vi "Global.vi"() -> ()   [LabVIEW 2020]
panel:
  in  "产品型号":string
  in  "结果显示字":refnum<vi>
  in  "前序状态显示字":refnum<vi>
  in  "前序状态":refnum<vi>
  in  "检测结果":refnum<vi>
  in  "合格数量":refnum<vi>
  in  "生产数量":refnum<vi>
  out "模式":u32
  in  "更换产品":refnum<vi>
  in  "提示信息":refnum<vi>
  in  "程序自动":refnum<vi>
  in  "报警图标":refnum<vi>
  in  "程序关闭":bool
  in  "Info":refnum<vi>
  in  "Result":refnum<vi>
  in  "批次":refnum<vi>
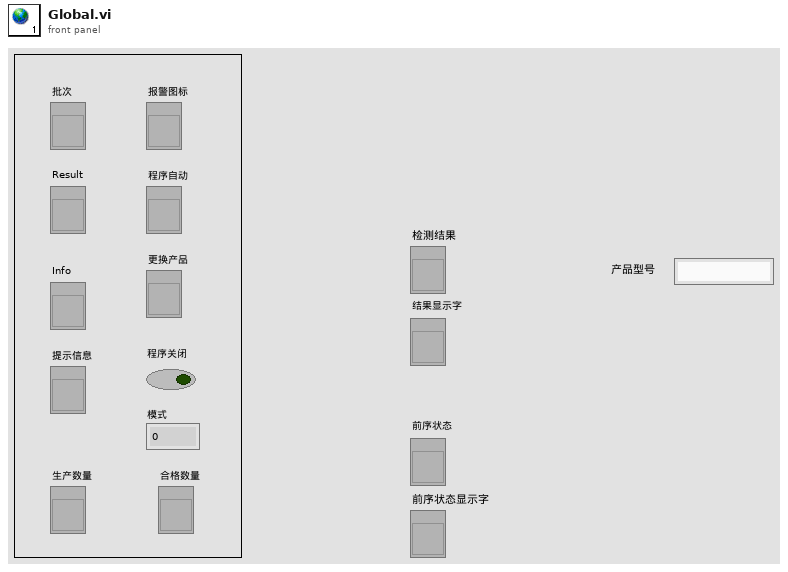
[diagram p1: front panel]
diagram:
